vi "DBL Complext From Items.vi"(10 "Level Items":T1[](array[typedef])) -> (2 "Array":cluster{dbl[]}[](array[cluster]))   [LabVIEW 2022 SP3]
uses:
  Ancestor Class/Front Panel Container/Tree/Tree/Type Def/Tree Item.ctl
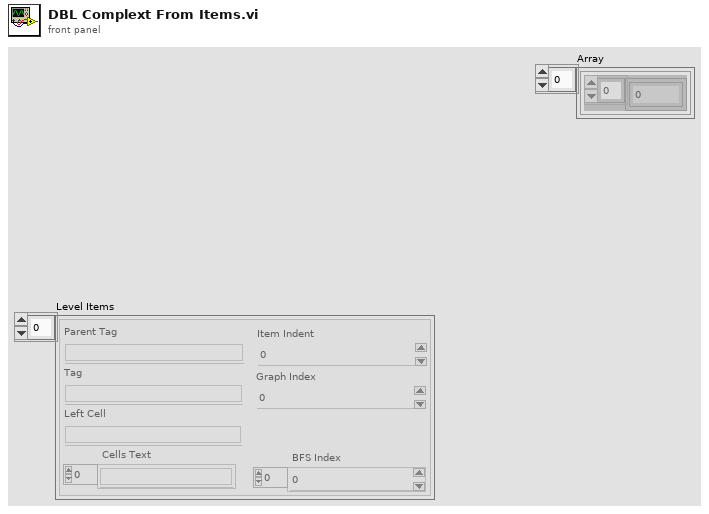
[diagram p1: front panel]
types:
  T1 = typedef "Tree Item.ctl" = cluster{"Parent Tag":string, "Tag":string, "Left Cell":string, "Cells Text":string[], "BFS Index":i32[], "Graph Index":i32, "Item Indent":i32}
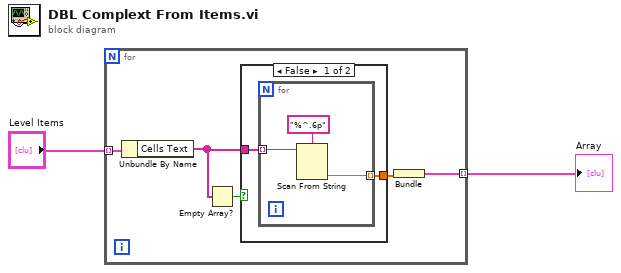
[diagram p0: block diagram]
diagram:
  n1 = for {
    tunnel: "Level Items" -> [w7] mode=indexing
    tunnel: [w5] -> w1 mode=indexing
    n2 = Unbundle By Name(w7) -> ("Cells Text"=w4:string[])
    n3 = Empty Array?(array=w4) -> (empty?=w3:bool)
    n4 = case shown="False" w3 {
      tunnel: [w9 _] -> w6
      tunnel: w4 -> [w8 _]
      frame False {
        n5 = for {
          tunnel: [w11] -> w9 mode=indexing
          tunnel: w8 -> [w10] mode=indexing
          n6 = Scan From String(format string="%^.6p", input string=w10) -> (output 1=w11:dbl)  [unwired: 3 in, 3 out]
        }
      }
      frame True {
      }
    }
    n7 = Bundle(w6) -> (w5:cluster{dbl[]})  [unwired: 1 in]
  }
  "Array" <- w1
